vi "Teleop.vi"(10 "Match Info":T1={"Autonomous Elapsed Seconds"=0.0, "TeleOp Elapsed Seconds"=0.0, "Disabled Elapsed Seconds"=0.0, "Visited Autonomous"=FALSE, "Visited TeleOp"=FALSE, "Visited Disabled"=FALSE, "Autonomous Settings"={"Autonomous Style"=enum."Independent", "VI Refnum"=refnum}}, 11 "Call Context":T2) -> ()   [LabVIEW 2019]
doc: "This VI is called for each enabled TeleOp packet received from the DS. It is typically used to read from joysticks and other inputs and update I/O or setpoints for timed control loops. It should complete and return within 20 milliseconds or risk missing DS packets."
uses:
  <vilib>/Rock Robotics/WPI/DriverStation/WPI_DriverStationDerivedRobotMode.ctl
  <vilib>/Rock Robotics/WPI/DriverStation/WPI_DriverStationMatch Info.ctl
  Framework/Robot Global Data.vi
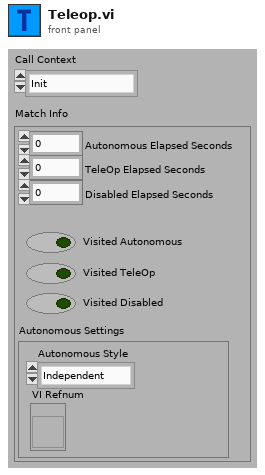
[diagram p1: front panel]
types:
  T1 = typedef "WPI_DriverStationMatch Info.ctl" = cluster{"Autonomous Elapsed Seconds":dbl, "TeleOp Elapsed Seconds":dbl, "Disabled Elapsed Seconds":dbl, "Visited Autonomous":bool, "Visited TeleOp":bool, "Visited Disabled":bool, "Autonomous Settings":cluster{"Autonomous Style":enum16{"Iterative", "Independent"}, "VI Refnum":refnum<vi>}}
  T2 = typedef "WPI_DriverStationDerivedRobotMode.ctl" = enum16{"Init", "Execute", "Stop"}
  T3 = typedef "Command Status Info.ctl" = cluster{"Name":string, "Status":T4, "notifier out":T5}
  T4 = typedef "Completion Status.ctl" = enum16{"Successful", "Aborted", "Incomplete"}
  T5 = typedef "Completion Notifier.ctl" = refnum<notifier>
  T6 = cluster{"XAngle":dbl, "YAngle":dbl, "ZAngle":dbl}
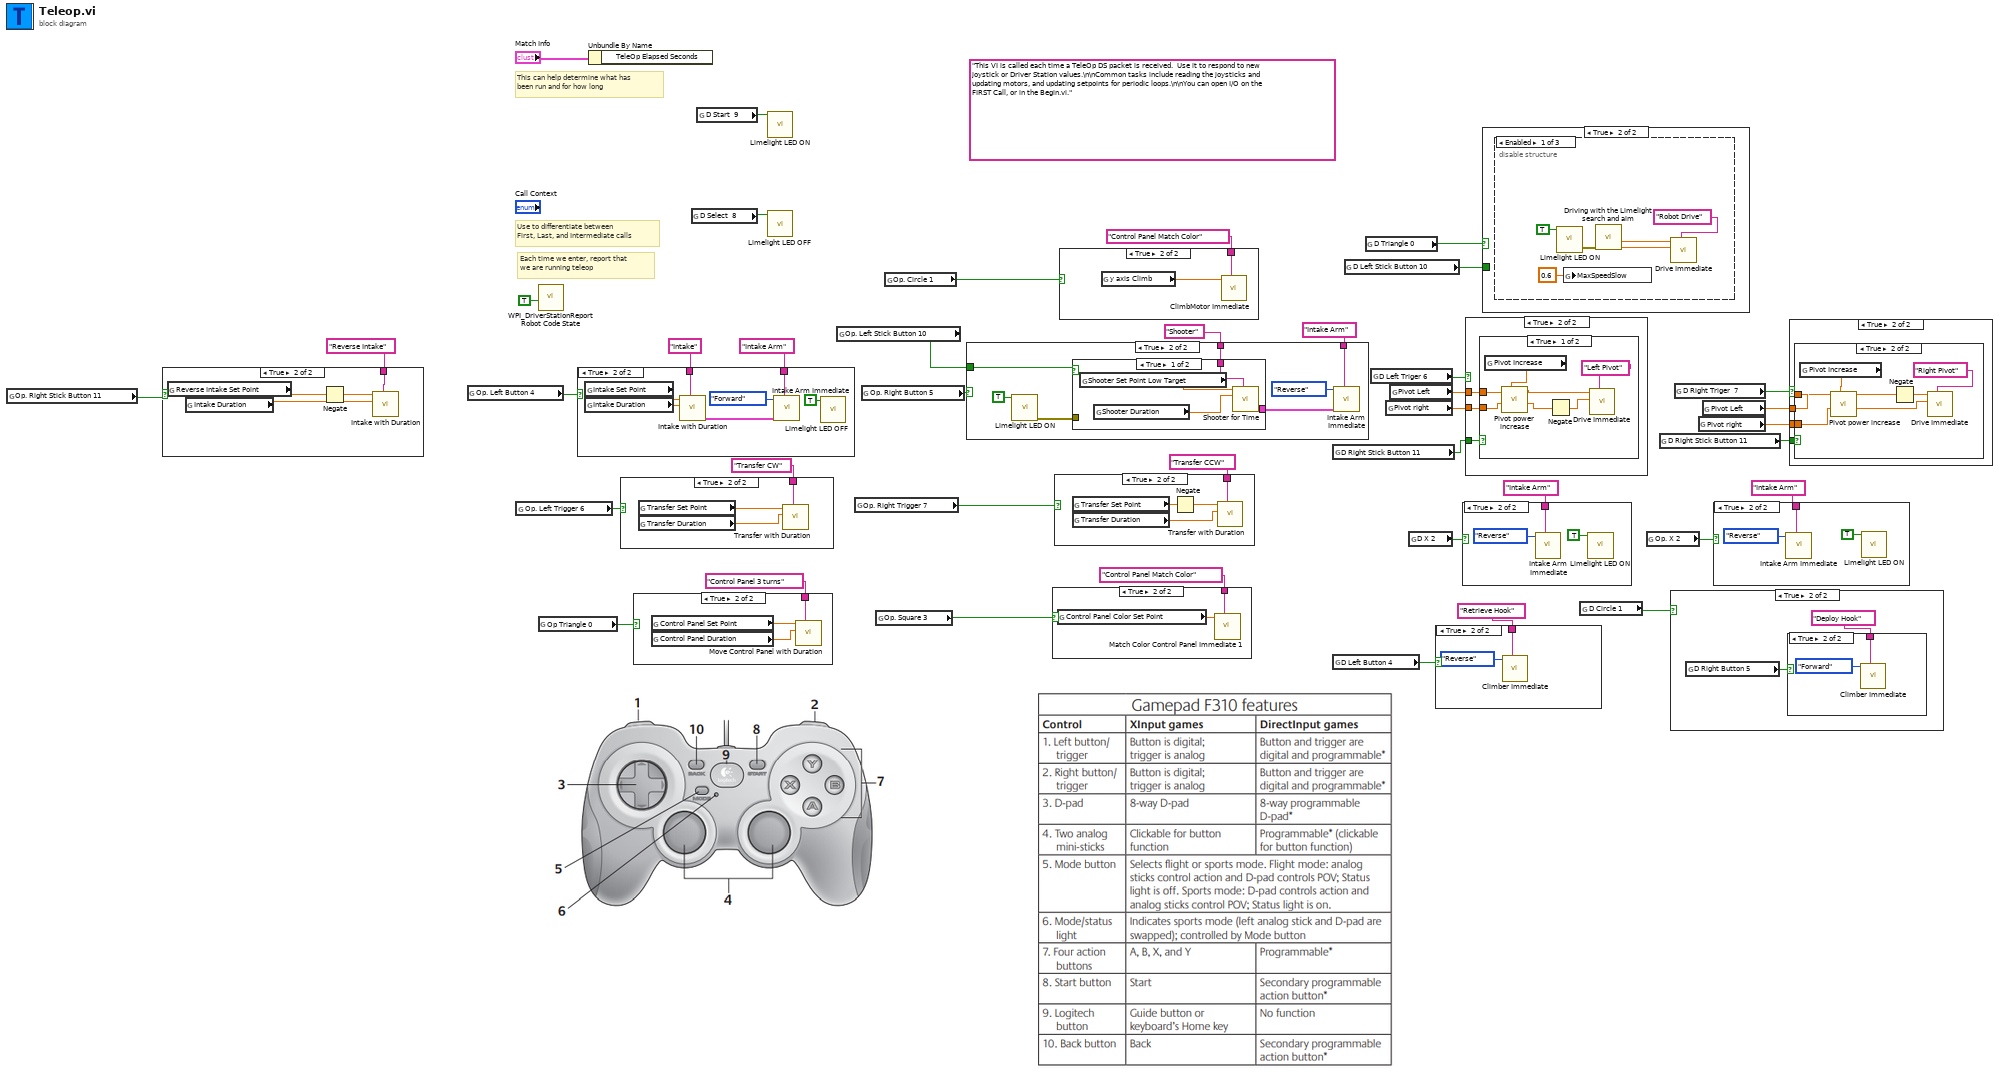
[diagram p0: block diagram]
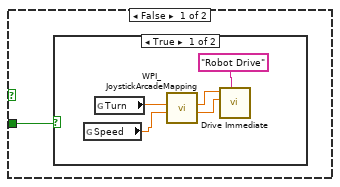
[diagram p8: hidden frame]
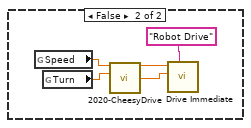
[diagram p9: hidden frame]
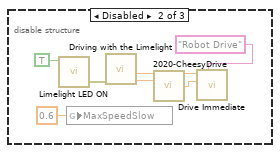
[diagram p10: hidden frame]
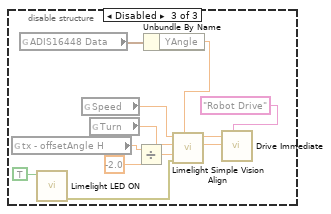
[diagram p11: hidden frame]
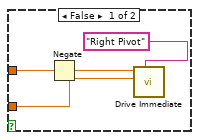
[diagram p16: hidden frame]
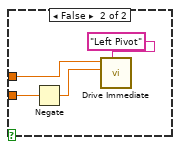
[diagram p18: hidden frame]
diagram:
  (unwired) "This VI is called each time a TeleOp DS packet is received.  Use it to respond to new joystick or Driver Station values.\n\nCommon tasks include reading the joysticks and updating motors, and updating setpoints for periodic loops.\n\nYou can open I/O on the FIRST Call, or in the Begin.vi."
  # "Each time we enter, report that\nwe are running teleop"
  # "Use to differentiate between\nFirst, Last, and Intermediate calls"
  # "This can help determine what has\nbeen run and for how long"
  n1 = global read "Robot Global Data.vi" "Op. Right Stick Button 11"() -> (w1:bool)
  n2 = case shown="True" w1 {
    tunnel: "Reverse Intake" ("refnum name") -> [_ w44]
    frame False {
    }
    frame True {
      n3 = global read "Robot Global Data.vi" "Reverse Intake Set Point"() -> (w43:dbl)
      n4 = global read "Robot Global Data.vi" "Intake Duration"() -> (w42:dbl)
      n5 = Negate(x=w43) -> (-x=w41:dbl)
      n6 = call "Intake with Duration.vi"("Description"=w44, "Duration (s)"=w42, "Setpoint"=w41) -> ()  [unwired: 8 in, 1 out]
    }
  }
  n7 = global read "Robot Global Data.vi" "Op. Left Button 4"() -> (w38:bool)
  n8 = global read "Robot Global Data.vi" "Op. Left Trigger 6"() -> (w32:bool)
  n9 = call <vilib>:"WPI_DriverStationReport Robot Code State.vi"("TeleOp"=TRUE ("Autonomous")) -> ()  [unwired: 10 in, 1 out]
  n10 = global read "Robot Global Data.vi" "Op Triangle 0"() -> (w25:bool)
  n11 = case shown="True" w38 {
    tunnel: "Intake" ("refnum name") -> [_ w51]
    tunnel: "Intake Arm" ("refnum name") -> [_ w47]
    frame False {
    }
    frame True {
      n12 = global read "Robot Global Data.vi" "Intake Set Point"() -> (w50:dbl)
      n13 = global read "Robot Global Data.vi" "Intake Duration"() -> (w49:dbl)
      n14 = call "Intake with Duration.vi"("Description"=w51, "Duration (s)"=w49, "Setpoint"=w50) -> ("Command Info Out"=w46:T3)  [unwired: 8 in]
      n15 = call "Intake Arm Immediate.vi"("Description"=w47, "Command Info In"=w46, "Relay Value"=enum16{"Off", "On", "Forward", "Reverse"}."Forward") -> ()  [unwired: 8 in, 1 out]
      n16 = call "Limelight LED OFF.vi"("D Select  8"=TRUE) -> ()  [unwired: 11 in]
    }
  }
  n17 = Unbundle By Name("Match Info") -> ()  [unwired: 1 out]
  n18 = case shown="True" w32 {
    tunnel: "Transfer CW" ("refnum name") -> [_ w54]
    frame False {
    }
    frame True {
      n19 = global read "Robot Global Data.vi" "Transfer Set Point"() -> (w53:dbl)
      n20 = global read "Robot Global Data.vi" "Transfer Duration"() -> (w52:dbl)
      n21 = call "Transfer with Duration.vi"("Description"=w54, "Duration (s)"=w52, "Setpoint"=w53) -> ()  [unwired: 8 in, 1 out]
    }
  }
  n22 = case shown="True" w25 {
    tunnel: "Control Panel 3 turns" ("refnum name") -> [_ w57]
    frame False {
    }
    frame True {
      n23 = global read "Robot Global Data.vi" "Control Panel Set Point"() -> (w56:dbl)
      n24 = global read "Robot Global Data.vi" "Control Panel Duration"() -> (w55:dbl)
      n25 = call "Move Control Panel with Duration.vi"("Description"=w57, "Duration (s)"=w55, "Setpoint"=w56) -> ()  [unwired: 8 in, 1 out]
    }
  }
  n26 = global read "Robot Global Data.vi" "D Select  8"() -> (w6:bool)
  n27 = global read "Robot Global Data.vi" "D Start  9"() -> (w7:bool)
  n28 = call "Limelight LED ON.vi"("D Start  9"=w7) -> ()  [unwired: 10 in, 1 out]
  n29 = call "Limelight LED OFF.vi"("D Select  8"=w6) -> ()  [unwired: 11 in]
  n30 = global read "Robot Global Data.vi" "Op. Left Stick Button 10"() -> (w8:bool)
  n31 = global read "Robot Global Data.vi" "Op. Right Trigger 7"() -> (w33:bool)
  n32 = global read "Robot Global Data.vi" "Op. Right Button 5"() -> (w34:bool)
  n33 = global read "Robot Global Data.vi" "Op. Square 3"() -> (w22:bool)
  n34 = global read "Robot Global Data.vi" "Op. Circle 1"() -> (w10:bool)
  n35 = case shown="True" w34 {
    tunnel: "Shooter" ("refnum name") -> [_ w64]
    tunnel: "Intake Arm" ("refnum name") -> [_ w62]
    tunnel: w8 -> [_ w60]
    frame False {
    }
    frame True {
      n36 = call "Limelight LED ON.vi"("D Start  9"=TRUE) -> ("error out"=w58:errorcluster)  [unwired: 10 in]
      n37 = case shown="True" w60 {
        tunnel: w64 -> [w68 w72]
        tunnel: [w65 w69] -> w61
        tunnel: w58 -> [_ _]
        frame True {
          n38 = global read "Robot Global Data.vi" "Shooter Set Point Low Target"() -> (w67:dbl)
          n39 = global read "Robot Global Data.vi" "Shooter Duration"() -> (w66:dbl)
          n40 = call "Shooter for Time.vi"("Description"=w68, "Duration (s)"=w66, "Setpoint"=w67) -> ("Command Info Out"=w65:T3)  [unwired: 8 in]
        }
        frame False {
          n41 = global read "Robot Global Data.vi" "Shooter Set Point"() -> (w71:dbl)
          n42 = global read "Robot Global Data.vi" "Shooter Duration"() -> (w70:dbl)
          n43 = call "Shooter for Time.vi"("Description"=w72, "Duration (s)"=w70, "Setpoint"=w71) -> ("Command Info Out"=w69:T3)  [unwired: 8 in]
        }
      }
      n44 = call "Intake Arm Immediate.vi"("Description"=w62, "Command Info In"=w61, "Relay Value"=enum16{"Off", "On", "Forward", "Reverse"}."Reverse") -> ()  [unwired: 8 in, 1 out]
    }
  }
  n45 = case shown="True" w22 {
    tunnel: "Control Panel Match Color" ("refnum name") -> [_ w74]
    frame False {
    }
    frame True {
      n46 = global read "Robot Global Data.vi" "Control Panel Color Set Point"() -> (w73:dbl)
      n47 = call "Match Color Control Panel Immediate 1.vi"("Description"=w74, "Setpoint"=w73) -> ()  [unwired: 9 in, 1 out]
    }
  }
  n48 = case shown="True" w33 {
    tunnel: "Transfer CCW" ("refnum name") -> [_ w78]
    frame False {
    }
    frame True {
      n49 = global read "Robot Global Data.vi" "Transfer Set Point"() -> (w76:dbl)
      n50 = global read "Robot Global Data.vi" "Transfer Duration"() -> (w75:dbl)
      n51 = Negate(x=w76) -> (-x=w77:dbl)
      n52 = call "Transfer with Duration.vi"("Description"=w78, "Duration (s)"=w75, "Setpoint"=w77) -> ()  [unwired: 8 in, 1 out]
    }
  }
  n53 = case shown="True" w10 {
    tunnel: "Control Panel Match Color" ("refnum name") -> [_ w80]
    frame False {
    }
    frame True {
      n54 = global read "Robot Global Data.vi" "y axis Climb"() -> (w79:dbl)
      n55 = call "ClimbMotor Immediate.vi"("Description"=w80, "Setpoint"=w79) -> ()  [unwired: 9 in, 1 out]
    }
  }
  n56 = global read "Robot Global Data.vi" "D Right Stick Button 11"() -> (w3:bool)
  n57 = global read "Robot Global Data.vi" "D Left Button 4"() -> (w15:bool)
  n58 = global read "Robot Global Data.vi" "D Left Stick Button 10"() -> (w5:bool)
  n59 = global read "Robot Global Data.vi" "D Triangle 0"() -> (w16:bool)
  n60 = global read "Robot Global Data.vi" "D Left Triger 6"() -> (w30:bool)
  n61 = global read "Robot Global Data.vi" "Pivot right"() -> (w19:dbl)
  n62 = global read "Robot Global Data.vi" "Pivot Left"() -> (w20:dbl)
  n63 = global read "Robot Global Data.vi" "D X 2"() -> (w23:bool)
  n64 = case shown="True" w15 {
    tunnel: "Retrieve Hook" ("refnum name") -> [_ w81]
    frame False {
    }
    frame True {
      n65 = call "Climber Immediate.vi"("Description"=w81, "Value"=enum16{"Off", "On", "Forward", "Reverse"}."Reverse" ("Relay Value")) -> ()  [unwired: 9 in, 1 out]
    }
  }
  n66 = case shown="True" w23 {
    tunnel: "Intake Arm" ("refnum name") -> [_ w84]
    frame False {
    }
    frame True {
      n67 = call "Intake Arm Immediate.vi"("Description"=w84, "Relay Value"=enum16{"Off", "On", "Forward", "Reverse"}."Reverse") -> ()  [unwired: 9 in, 1 out]
      n68 = call "Limelight LED ON.vi"("D Start  9"=TRUE) -> ()  [unwired: 10 in, 1 out]
    }
  }
  n69 = case shown="True" w30 {
    tunnel: w20 -> [_ w88]
    tunnel: w19 -> [_ w87]
    tunnel: w3 -> [_ w86]
    frame False {
    }
    frame True {
      n70 = case shown="True" w86 {
        tunnel: w88 -> [w93 w98]
        tunnel: w87 -> [w92 w97]
        frame True {
          n71 = global read "Robot Global Data.vi" "Pivot Increase"() -> (w89:dbl)
          n72 = call "Pivot power increase.vi"("Pivot Increase"=w89, "Input Pivot Right"=w92, "Input Pivot Left"=w93) -> ("Output Pivot Right"=w90:dbl, "Output Pivot Left"=w91:dbl)  [unwired: 7 in]
          n73 = Negate(x=w90) -> (-x=w94:dbl)
          n74 = call "Drive Immediate.vi"("Description"="Left Pivot", "Right Setpoint"=w94, "Left Setpoint"=w91) -> ()  [unwired: 8 in, 1 out]
        }
        frame False {
          n75 = Negate(x=w97) -> (-x=w96:dbl)
          n76 = call "Drive Immediate.vi"("Description"="Left Pivot", "Right Setpoint"=w96, "Left Setpoint"=w98) -> ()  [unwired: 8 in, 1 out]
        }
      }
    }
  }
  n77 = case shown="True" w16 {
    tunnel: w5 -> [w100 _]
    frame False {
      n78 = case shown="True" w100 {
        frame True {
          n79 = global read "Robot Global Data.vi" "Speed"() -> (w103:dbl)
          n80 = global read "Robot Global Data.vi" "Turn"() -> (w104:dbl)
          n81 = call <vilib>:"WPI_JoystickArcadeMapping.vi"("Y axis value"=w103, "X axis value"=w104) -> ("Right Motor Value"=w101:dbl, "Left Motor Value"=w102:dbl)  [unwired: 8 in]
          n82 = call "Drive Immediate.vi"("Description"="Robot Drive", "Right Setpoint"=w101, "Left Setpoint"=w102) -> ()  [unwired: 8 in, 1 out]
        }
        frame False {
          n83 = global read "Robot Global Data.vi" "Speed"() -> (w107:dbl)
          n84 = global read "Robot Global Data.vi" "Turn"() -> (w108:dbl)
          n85 = call "2020-CheesyDrive.vi"("Throttle"=w107, "Wheel"=w108) -> ("Left PWM"=w109:dbl, "Right PWM"=w110:dbl)  [unwired: 12 in]
          n86 = call "Drive Immediate.vi"("Description"="Robot Drive", "Right Setpoint"=w110, "Left Setpoint"=w109) -> ()  [unwired: 8 in, 1 out]
        }
      }
    }
    frame True {
      n87 = disable-structure shown="Enabled" {
        frame Enabled {
          n88 = call "Limelight LED ON.vi"("D Start  9"=TRUE) -> ("error out"=w115:errorcluster)  [unwired: 10 in]
          n89 = global write "Robot Global Data.vi" "MaxSpeedSlow"(0.6 ("MaxSpeedSlow")) -> ()
          n90 = call "Driving with the Limelight search and aim.vi"("error in (no error)"=w115) -> ("TurnCommand"=w111:dbl, "SpeedCommand"=w112:dbl)  [unwired: 8 in, 1 out]
          n91 = call "Drive Immediate.vi"("Description"="Robot Drive", "Right Setpoint"=w111, "Left Setpoint"=w112) -> ()  [unwired: 8 in, 1 out]
        }
        frame Disabled {
          n92 = call "Limelight LED ON.vi"("D Start  9"=TRUE) -> ("error out"=w119:errorcluster)  [unwired: 10 in]
          n93 = global write "Robot Global Data.vi" "MaxSpeedSlow"(0.6 ("MaxSpeedSlow")) -> ()
          n94 = call "Driving with the Limelight.vi"("error in (no error)"=w119) -> ("TurnCommand"=w120:dbl, "SpeedCommand"=w121:dbl)  [unwired: 8 in, 1 out]
          n95 = call "2020-CheesyDrive.vi"("Throttle"=w121, "Wheel"=w120) -> ("Left PWM"=w123:dbl, "Right PWM"=w124:dbl)  [unwired: 12 in]
          n96 = call "Drive Immediate.vi"("Description"="Robot Drive", "Right Setpoint"=w124, "Left Setpoint"=w123) -> ()  [unwired: 8 in, 1 out]
        }
        frame Disabled {
          n97 = global read "Robot Global Data.vi" "tx - offsetAngle H"() -> (w130:dbl)
          n98 = global read "Robot Global Data.vi" "ADIS16448 Data"() -> (w126:T6)
          n99 = call "Limelight LED ON.vi"("D Start  9"=TRUE) -> ("error out"=w134:errorcluster)  [unwired: 10 in]
          n100 = global read "Robot Global Data.vi" "Speed"() -> (w128:dbl)
          n101 = global read "Robot Global Data.vi" "Turn"() -> (w127:dbl)
          n102 = Divide(x=w130, y=-2.0) -> (x/y=w131:dbl)
          n103 = Unbundle By Name(w126) -> ("YAngle"=w125:dbl)
          n104 = call "Limelight Simple Vision Align.vi"("Gyro Angle"=w125, "error in (no error)"=w134, "Target Offset"=w131, "Manual Turn"=w127, "Throttle"=w128) -> ("Right Power"=w132:dbl, "Left Power"=w133:dbl)  [unwired: 5 in]
          n105 = call "Drive Immediate.vi"("Description"="Robot Drive", "Right Setpoint"=w132, "Left Setpoint"=w133) -> ()  [unwired: 8 in, 1 out]
        }
      }
    }
  }
  n106 = global read "Robot Global Data.vi" "D Circle 1"() -> (w9:bool)
  n107 = global read "Robot Global Data.vi" "Op. X 2"() -> (w13:bool)
  n108 = global read "Robot Global Data.vi" "D Right Stick Button 11"() -> (w4:bool)
  n109 = case shown="True" w9 {
    frame False {
    }
    frame True {
      n110 = global read "Robot Global Data.vi" "D Right Button 5"() -> (w137:bool)
      n111 = case shown="True" w137 {
        tunnel: "Deploy Hook" ("refnum name") -> [_ w139]
        frame False {
        }
        frame True {
          n112 = call "Climber Immediate.vi"("Description"=w139, "Value"=enum16{"Off", "On", "Forward", "Reverse"}."Forward" ("Relay Value")) -> ()  [unwired: 9 in, 1 out]
        }
      }
    }
  }
  n113 = global read "Robot Global Data.vi" "D Right Triger  7"() -> (w29:bool)
  n114 = global read "Robot Global Data.vi" "Pivot right"() -> (w17:dbl)
  n115 = global read "Robot Global Data.vi" "Pivot Left"() -> (w18:dbl)
  n116 = case shown="True" w13 {
    tunnel: "Intake Arm" ("refnum name") -> [_ w142]
    frame False {
    }
    frame True {
      n117 = call "Intake Arm Immediate.vi"("Description"=w142, "Relay Value"=enum16{"Off", "On", "Forward", "Reverse"}."Reverse") -> ()  [unwired: 9 in, 1 out]
      n118 = call "Limelight LED ON.vi"("D Start  9"=TRUE) -> ()  [unwired: 10 in, 1 out]
    }
  }
  n119 = case shown="True" w29 {
    tunnel: w18 -> [_ w146]
    tunnel: w17 -> [_ w145]
    tunnel: w4 -> [_ w144]
    frame False {
    }
    frame True {
      n120 = case shown="True" w144 {
        tunnel: w146 -> [w149 w155]
        tunnel: w145 -> [w148 w154]
        frame False {
          n121 = Negate(x=w149) -> (-x=w147:dbl)
          n122 = call "Drive Immediate.vi"("Description"="Right Pivot", "Right Setpoint"=w148, "Left Setpoint"=w147) -> ()  [unwired: 8 in, 1 out]
        }
        frame True {
          n123 = global read "Robot Global Data.vi" "Pivot Increase"() -> (w151:dbl)
          n124 = call "Pivot power increase.vi"("Pivot Increase"=w151, "Input Pivot Right"=w154, "Input Pivot Left"=w155) -> ("Output Pivot Right"=w152:dbl, "Output Pivot Left"=w153:dbl)  [unwired: 7 in]
          n125 = Negate(x=w153) -> (-x=w156:dbl)
          n126 = call "Drive Immediate.vi"("Description"="Right Pivot", "Right Setpoint"=w152, "Left Setpoint"=w156) -> ()  [unwired: 8 in, 1 out]
        }
      }
    }
  }
